vi "delete from array.vi"(8 "index":i32, 11 "array in":string[](array[string])) -> (3 "array out":string[](array[string]))   [LabVIEW 2024, in "summary manager.lvlib"]
uses:
  summary manager.lvlib
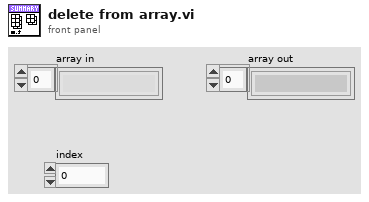
[diagram p1: front panel]
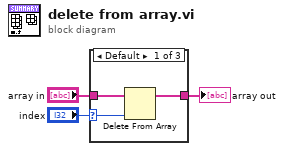
[diagram p0: block diagram]
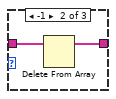
[diagram p2: hidden frame]
diagram:
  n1 = case shown="Default" "index" {
    selector: "index" -> [w4 _ _]
    tunnel: [w5 w8 _] -> w3
    tunnel: "array in" -> [w6 w7 _]
    frame Default {
      n2 = Delete From Array(array=w6, index=w4) -> (array with subset deleted=w5:string[])  [unwired: 1 in, 1 out]
    }
    frame -1 {
      n3 = Delete From Array(array=w7) -> (array with subset deleted=w8:string[])  [unwired: 2 in, 1 out]
    }
    frame -2 {
    }
  }
  "array out" <- w3
